vi "CameraStartAcquire.vi"(8 "error in (no error)":errorcluster, 11 "CameraBase in":refnum<class "CameraBase.lvclass">) -> (0 "error out":errorcluster, 3 "CameraBase out":refnum<class "CameraBase.lvclass">)   [LabVIEW 2010, in "CameraBase.lvclass"]
uses:
  CameraBase.lvclass
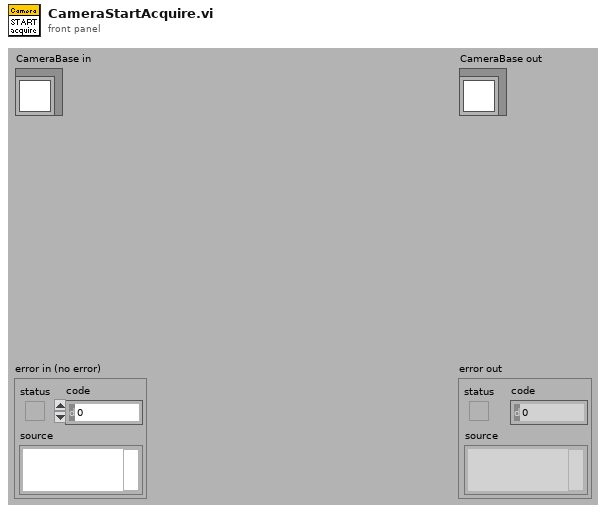
[diagram p1: front panel]
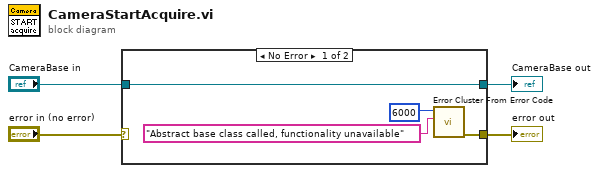
[diagram p0: block diagram]
diagram:
  n1 = case shown="No Error" "error in (no error)" {
    selector: "error in (no error)" -> [_ w10]
    tunnel: [w7 w10] -> w3
    tunnel: [w5 w9] -> w1
    tunnel: "CameraBase in" -> [w5 w9]
    frame No Error {
      n2 = call <vilib>:"Error Cluster From Error Code.vi"("error message (\"\")"="Abstract base class called, functionality unavailable" ("format string"), "error code (0)"=6000) -> ("error out"=w7:errorcluster)  [unwired: 7 in]
    }
    frame Error {
    }
  }
  "error out" <- w3
  "CameraBase out" <- w1
